vi "UTS - Parse Response String.vi"(8 "error in (no error)":errorcluster, 10 "Response String in":string, 11 "Return Request in":T1) -> (0 "error out":errorcluster, 2 "Response String out":string, 3 "Return Request out":T1)   [LabVIEW 2017, in "SSH.lvlib"]
uses:
  SSH.lvlib
  Return Request Configuration.ctl
  Response Configuration.ctl
  Expected Response String Config.ctl
  Search Start Point.ctl
  Character Count Configuration.ctl
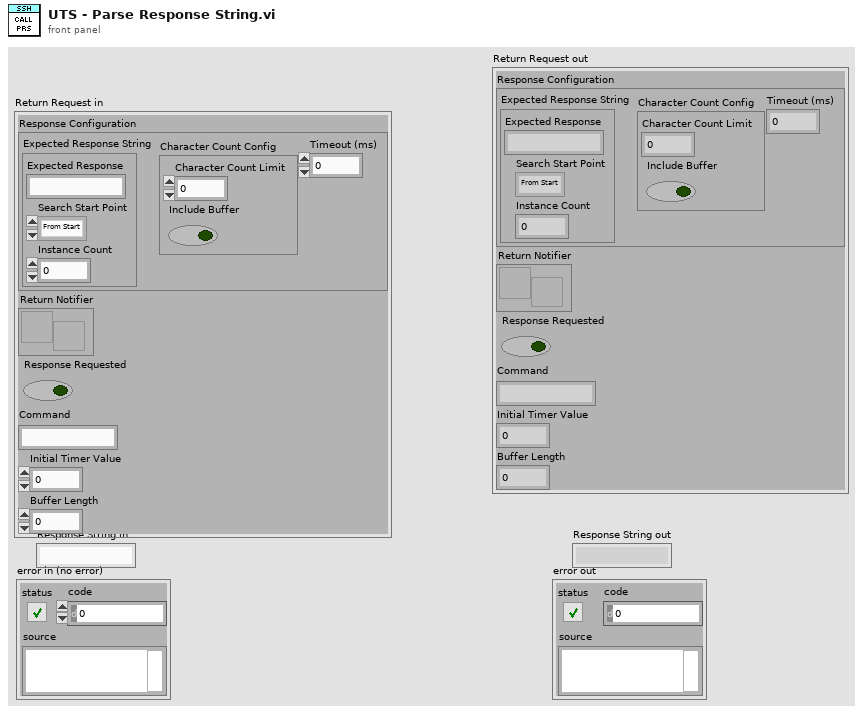
[diagram p1: front panel]
types:
  T1 = typedef "SSH.lvlib/Return Request Configuration.ctl" = cluster{"Response Configuration":T2, "Return Notifier":refnum<notifier>, "Response Requested":bool, "Command":string, "Initial Timer Value":u32, "Buffer Length":i32}
  T2 = typedef "SSH.lvlib/Response Configuration.ctl" = cluster{"Expected Response String":T3, "Character Count Config":T5, "Timeout (ms)":i32}
  T3 = typedef "SSH.lvlib/Expected Response String Config.ctl" = cluster{"Expected Response":string, "Search Start Point":T4, "Instance Count":i32}
  T4 = typedef "SSH.lvlib/Search Start Point.ctl" = enum16{"From Start", "From End"}
  T5 = typedef "SSH.lvlib/Character Count Configuration.ctl" = cluster{"Character Count Limit":i32, "Include Buffer":bool}
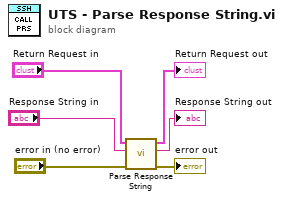
[diagram p0: block diagram]
diagram:
  n1 = call "Parse Response String.vi"("error in (no error)"="error in (no error)", "Response String in"="Response String in", "Return Request in"="Return Request in") -> ("error out"=→"error out":errorcluster, "Response String out"=→"Response String out":string, "Return Request out"=→"Return Request out":T1)  [unwired: 6 in]
